vi "Shell32.ShellExecuteA.vi"(0 "path":path=path "C:/Users/Frederic Schmitt/Desktop/GE/Sciospec Bioimpedance - Sinan/Sciospec ISX3v2/Sciospec_ISX3v2_201902_04.jar", 11 "error in (no error)":errorcluster) -> (15 "error out":errorcluster)   [LabVIEW 2012]
uses:
  shell32.dll
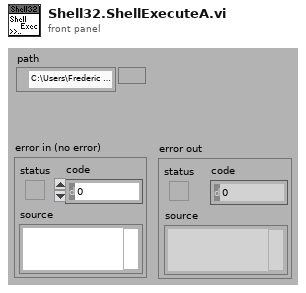
[diagram p1: front panel]
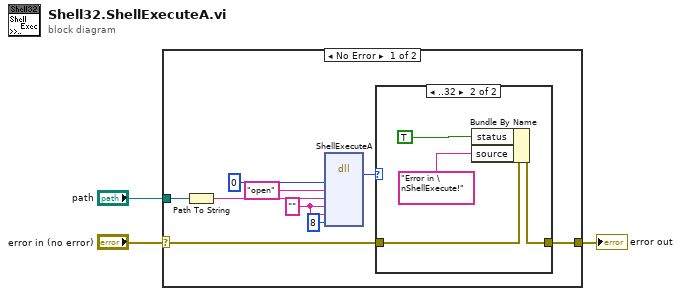
[diagram p0: block diagram]
diagram:
  n1 = case shown="No Error" "error in (no error)" {
    selector: "error in (no error)" -> [w5 w18]
    tunnel: "path" -> [w10 _]
    tunnel: [w4 w18] -> w1
    frame No Error {
      w8 = "" ("lpParameters")
      n2 = Path To String(path=w10) -> (string=w9:string)
      n3 = dll-call lib="shell32.dll" fn="ShellExecuteA"("hwnd"=0, "lpOperation"="open", "lpFile"=w9, "lpParameters"=w8, "lpDirectory"=w8, "nShowCmd"=8) -> (w6:i32)  [unwired: 9 in, 2 out]
      n4 = case shown="..32" w6 {
        tunnel: w5 -> [w13 w17]
        tunnel: [w13 w15] -> w4
        frame Default {
        }
        frame ..32 {
          n5 = Bundle By Name(cluster=w17, "status"=TRUE, "source"="Error in \nShellExecute!") -> (w15:errorcluster)
        }
      }
    }
    frame Error {
    }
  }
  "error out" <- w1
